vi "Create Mapping.vi"(10 "Channels In":refnum<class "TBM channel.lvclass">[](array[class]), 11 "Data Dictionary In":refnum<class "data dictionary.lvclass">) -> (3 "Array out":T1[](array[typedef]))   [LabVIEW 2013, in "J1939 runtime.lvclass"]
uses:
  J1939 runtime.lvclass
  configuration/Signal Mapping.ctl
  <vilib>/NI/Tag Bus/tag/Data Type.ctl
  <vilib>/NI/Tag Bus Module Framework/channel/TBM channel.lvclass
  <vilib>/NI/Tag Bus/dictionary/data dictionary.lvclass
  <vilib>/NI/Tag Bus/tag/tag descriptor.lvclass/tag descriptor.ctl
  <vilib>/NI/Tag Bus/tag/read tag name.vi
  <vilib>/NI/Tag Bus/dictionary/locate tag.vi
  <vilib>/NI/Tag Bus/tag/tag descriptor.lvclass
  configuration/J1939 configuration.lvclass
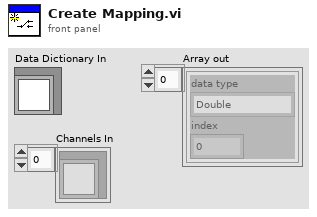
[diagram p1: front panel]
types:
  T1 = typedef "J1939 configuration.lvclass/Signal Mapping.ctl" = cluster{"data type":T2, "index":i32}
  T2 = typedef "tag bus.lvlib/tag descriptor.lvclass/Data Type.ctl" = enum16{"Double", "Single", "I64", "I32", "I16", "I8", "U64", "U32", "U16", "U8", "Boolean", "String", "Array of Double", "Array of Single", "Array of I64", "Array of I32", "Array of I16", "Array of I8", "Array of U64", "Array of U32", "Array of U16", "Array of U8", "Array of Boolean", "Array of String"}
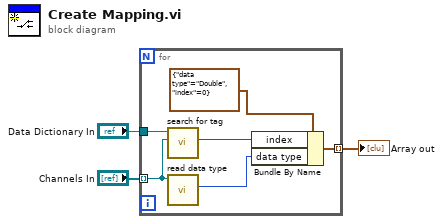
[diagram p0: block diagram]
diagram:
  n1 = for {
    tunnel: "Data Dictionary In" -> [w9]
    tunnel: "Channels In" -> [w5] mode=indexing
    tunnel: [w7] -> w3 mode=indexing
    n2 = call <vilib>:"search for tag.vi"("system tag"=w5, "data dictionary in"=w9) -> ("index"=w6:i32)  [unwired: 7 in, 2 out]
    n3 = call <vilib>:"read data type.vi"("system tag in"=w5) -> ("data type"=w4:T2)  [unwired: 8 in, 2 out]
    n4 = Bundle By Name(cluster=T1 {"data type"=enum."Double", "index"=0}, "index"=w6, "data type"=w4) -> (w7:T1)
  }
  "Array out" <- w3
